vi "DELETE Save Directory.vi"   [LabVIEW 2013]
uses:
  Action.ctl
  Persistent Data FGV Selector.ctl
types:
  T1 = typedef "Persistent Data FGV Selector.ctl" = enum16{"Save Directory", "File Name"}
  T2 = typedef "Action.ctl" = enum16{"GET", "PUT", "DELETE"}
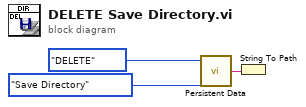
[diagram p0: block diagram]
diagram:
  n1 = call "Persistent Data.vi"("Persistent Data FGV Selector"=Persistent_Data_FGV_Selector."Save Directory", "Action"=Action."DELETE") -> ("Output"=w1:string)  [unwired: 1 in]
  n2 = String To Path(string=w1) -> ()  [unwired: 1 out]
